vi "DestroyMonitor.vi"(8 "Error In":errorcluster, 11 "Handle in":i32) -> (0 "Error Out":errorcluster)   [LabVIEW 2016]
uses:
  kernel32.dll
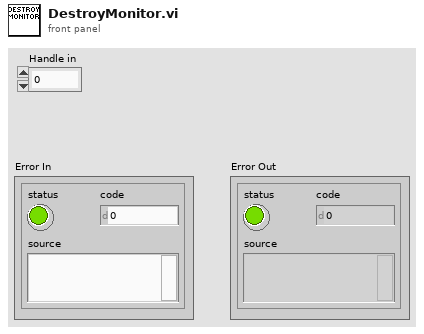
[diagram p1: front panel]
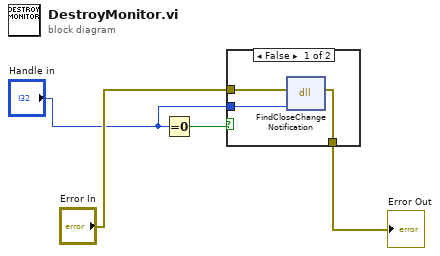
[diagram p0: block diagram]
diagram:
  n1 = Equal To 0?(x="Handle in") -> (x = 0?=w2:bool)
  n2 = case shown="False" w2 {
    tunnel: "Error In" -> [w7 w8]
    tunnel: [w6 w8] -> w3
    tunnel: "Handle in" -> [w5 _]
    frame False {
      n3 = dll-call lib="kernel32.dll" fn="FindCloseChangeNotification"(error in=w7, "Handle"=w5) -> (error out=w6:errorcluster)  [unwired: 4 in, 1 out]
    }
    frame True {
    }
  }
  "Error Out" <- w3
